vi "NI VeriStand - Visually Update the System Explorer Tree.vi"(8 "error in (no error)":errorcluster, 11 "Node IDs":u64[](array[numeric])) -> (0 "error out":errorcluster)   [LabVIEW 2016, in "Ballard Arinc-429 System Explorer.lvlib"]
doc: "***This VI is not officially supported by National Instruments*** due to CAR 317524"
uses:
  Ballard Arinc-429 System Explorer.lvlib
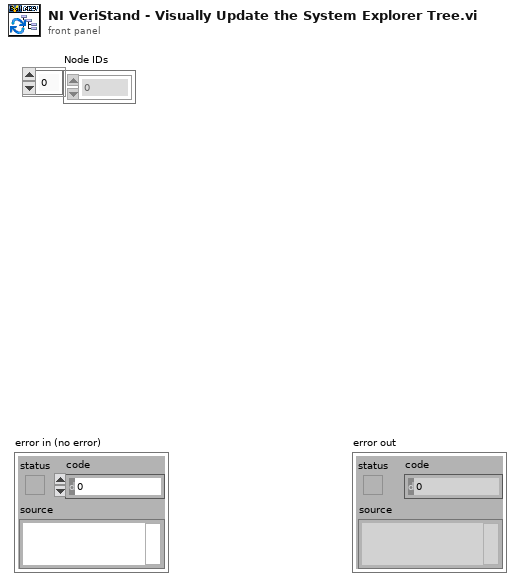
[diagram p1: front panel]
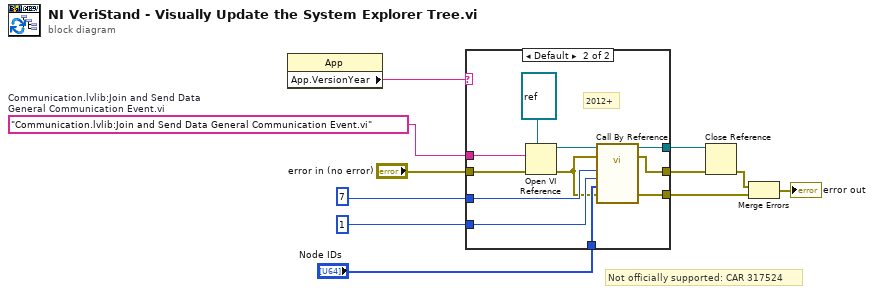
[diagram p0: block diagram]
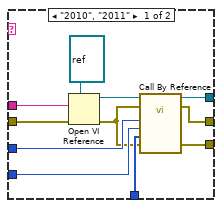
[diagram p2: hidden frame]
diagram:
  w11 = "Communication.lvlib:Join and Send Data General Communication Event.vi"  # Communication.lvlib:Join and Send Data General Communication Event.vi
  # "Not officially supported: CAR 317524"
  n1 = property class="App"() -> ("App.VersionYear"=w1:string)  [unwired: 2 in, 2 out]
  n2 = case shown="Default" w1 {
    tunnel: w11 -> [w22 w33]
    tunnel: "error in (no error)" -> [w21 w32]
    tunnel: 7 -> [w18 w30]
    tunnel: 1 -> [w17 w29]
    tunnel: "Node IDs" -> [w16 w28]
    tunnel: [w14 w26] -> w5
    tunnel: [w13 w25] -> w4
    tunnel: [w12 w24] -> w2
    frame "2010", "2011" {
      n3 = Open VI Reference(type specifier VI Refnum (for type only)=refnum<vi> refnum, vi path=w22, error in (no error)=w21) -> (vi reference=w19:refnum<vi>, error out=w15:errorcluster)  [unwired: 3 in]
      n4 = call-by-ref "?"(reference=w19, error in=w15, 8:"error in (no error)"=w15, "Data in"=w16, "Listener"=w17, "Action"=w18) -> (reference out=w13:refnum<vi>, error out=w14:errorcluster, 0:"error out"=w12:errorcluster)  [unwired: 6 in, 1 out]
    }
    frame Default {
      # "2012+"
      n5 = Open VI Reference(type specifier VI Refnum (for type only)=refnum<vi> refnum, vi path=w33, error in (no error)=w32) -> (vi reference=w31:refnum<vi>, error out=w27:errorcluster)  [unwired: 3 in]
      n6 = call-by-ref "?"(reference=w31, error in=w27, 8:"error in (no error)"=w27, "Data in"=w28, "Listener"=w29, "Action"=w30) -> (reference out=w25:refnum<vi>, error out=w26:errorcluster, 0:"error out"=w24:errorcluster)  [unwired: 6 in, 1 out]
    }
  }
  n7 = Close Reference(reference=w4, error in (no error)=w5) -> (error out=w3:errorcluster)
  n8 = Merge Errors(w3, w2) -> (→"error out":errorcluster)
